vi "retrieveJobClassInstance.vi"(8 "error in (no error)":errorcluster, 11 "VI in":refnum<vi>) -> (0 "error out":errorcluster, 1 "found":bool, 2 "Job":refnum<class "Job.lvclass">, 3 "VI out":refnum<vi>)   [LabVIEW 2013, in "openCronJob.lvlib" / "Job.StaticVIRef.lvclass"]
uses:
  Job.StaticVIRef.lvclass
  Job/Job.lvclass
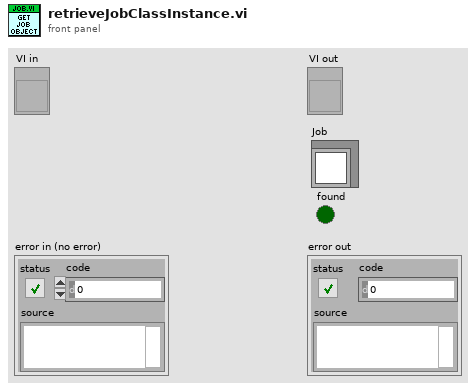
[diagram p1: front panel]
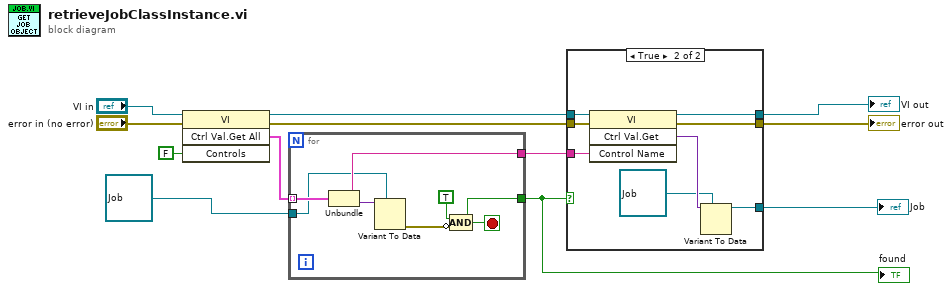
[diagram p0: block diagram]
diagram:
  n1 = invoke class="VI" method="Ctrl Val.Get All"(reference="VI in", error in="error in (no error)", "Controls"=FALSE) -> (reference out=w8:refnum<vi>, error out=w6:errorcluster, "Get All Control Values Variant"=w5:cluster{"Name":string, "Variant Data":variant}[])  [unwired: 1 in, 1 out]
  n2 = for {
    tunnel: w5 -> [w19] mode=indexing
    tunnel: refnum<class "Job.lvclass"> refnum ("openCronJob.lvlib:Job.lvclass") -> [w14]
    tunnel: [w16] -> w4
    tunnel: [w15] -> w3
    stop <- w16 stop-if-true
    n3 = Unbundle(w19) -> ("Name"=w15:string, "Variant Data"=w18:variant)
    n4 = Variant To Data(type=w14, Variant=w18) -> (error out=w17:errorcluster)  [unwired: 1 in, 1 out]
    n5 = Compound Arithmetic op=AND(TRUE, invert w17) -> (w16:bool)
  }
  "found" <- w4
  n6 = case shown="True" w4 {
    tunnel: [w20 w29] -> w12
    tunnel: [w21 w28] -> w11
    tunnel: w8 -> [w21 w27]
    tunnel: w6 -> [w20 w26]
    tunnel: [_ w22] -> w1
    tunnel: w3 -> [_ w25]
    frame False {
    }
    frame True {
      n7 = invoke class="VI" method="Ctrl Val.Get"(reference=w27, error in=w26, "Control Name"=w25) -> (reference out=w28:refnum<vi>, error out=w29:errorcluster, "Get Control Value Variant"=w24:variant)  [unwired: 1 in, 1 out]
      n8 = Variant To Data(type=refnum<class "Job.lvclass"> refnum ("openCronJob.lvlib:Job.lvclass"), Variant=w24) -> (data=w22:refnum<class "Job.lvclass">)  [unwired: 1 in, 1 out]
    }
  }
  "error out" <- w12
  "VI out" <- w11
  "Job" <- w1
